vi "lfield_write_is_visible.vi"(8 "error in (no error)":errorcluster, 10 "Is Visible?":bool=TRUE, 11 "lightfield_class in":refnum<class "lightfield_class.lvclass">) -> (0 "error out":errorcluster, 3 "lightfield_class out":refnum<class "lightfield_class.lvclass">)   [LabVIEW 2015, in "lightfield_class.lvclass"]
uses:
  lightfield_class.lvclass
  lightfield_class.lvclass/lightfield_class.ctl
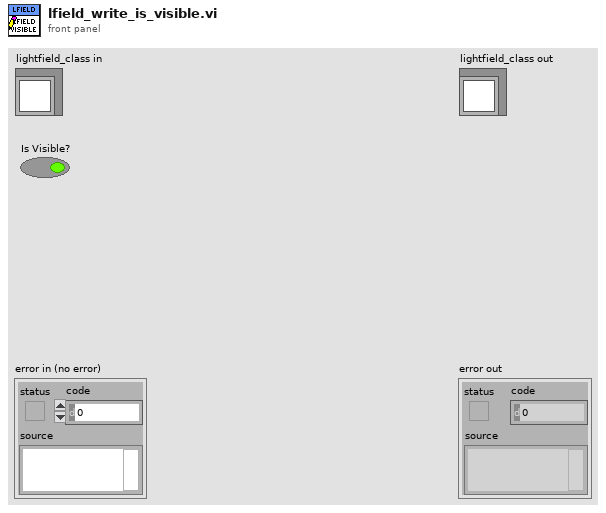
[diagram p1: front panel]
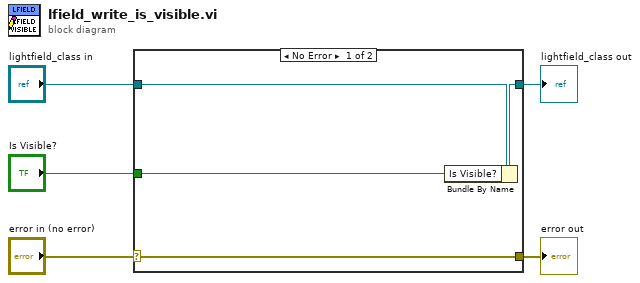
[diagram p0: block diagram]
diagram:
  n1 = case shown="No Error" "error in (no error)" {
    selector: "error in (no error)" -> [w9 w10]
    tunnel: [w9 w10] -> w4
    tunnel: [w7 w11] -> w2
    tunnel: "lightfield_class in" -> [w8 w11]
    tunnel: "Is Visible?" -> [w6 _]
    frame No Error {
      n2 = Bundle By Name(cluster=w8, "Is Visible?"=w6) -> (w7:refnum<class "lightfield_class.lvclass">)
    }
    frame Error {
    }
  }
  "error out" <- w4
  "lightfield_class out" <- w2
